vi "FitToolingPinImage.vi"(7 "Pattern Match Settings":T4={"Algorithm"=2, "Number of Matches Requested"=1, "Minimum Match Score"=700.0, "SubPixel Accuracy"=TRUE, "Rotation Angle Ranges"=[{"Start"=-90.0, "End"=90.0}], "Show Search Area"=FALSE, "Show Result"=TRUE} {"Rotation Angle Ranges"."End" format="%.1f"; "Rotation Angle Ranges"."Start" format="%.1f"; "Minimum Match Score" min=0 max=1000 format="%.2f"; "Number of Matches Requested" min=1; "Algorithm" items=["All", "Low Discrepancy Sampling", "Grayscale Value Pyramid", "Gradients Pyramid"]}, 9 "Calibrated Image":T1, 10 "Search Rect":T3={"Left"=0, "Top"=0, "Right"=2147483647, "Bottom"=2147483647, "Rotation"=0.0} {"Rotation" format="%.2f"; "Left" scale=0.0..1024.0; "Right" scale=0.0..1024.0}, 11 "Template":T1) -> (1 "Corner positions":sgl[](array[numeric]), 3 "Refnum out":T1)   [LabVIEW 2016]
uses:
  <vilib>/vision/Image Controls.llb/IMAQ Image.ctl
  <vilib>/vision/NI_Vision_Development_Module.lvlib
panel:
  out "Matches (pixel)":T2(array[cluster]) {"Bounding Box"."y" format="%.2f"; "Bounding Box"."x" format="%.2f"; "Position"."y" format="%.2f"; "Position"."x" format="%.2f"; "Score" format="%.2f"; "Scale" format="%.2f"; "Angle" format="%.2f"}
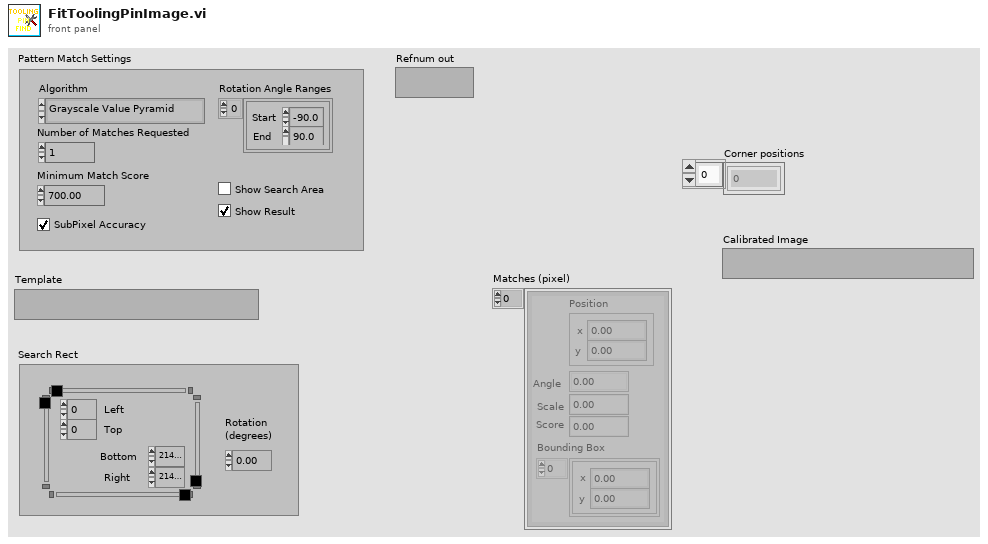
[diagram p1: front panel]
types:
  T1 = typedef "IMAQ Image.ctl" = refnum<image>
  T2 = cluster{"Position":cluster{"x":sgl, "y":sgl}, "Angle":sgl, "Scale":sgl, "Score":sgl, "Bounding Box":cluster{"x":sgl, "y":sgl}[]}[]
  T3 = typedef "IMAQ Rectangle" = cluster{"Left":i32, "Top":i32, "Right":i32, "Bottom":i32, "Rotation":dbl}
  T4 = cluster{"Algorithm":i32, "Number of Matches Requested":i32, "Minimum Match Score":sgl, "SubPixel Accuracy":bool, "Rotation Angle Ranges":cluster{"Start":sgl, "End":sgl}[], "Show Search Area":bool, "Show Result":bool}
  T5 = cluster{"Left":i32, "Top":i32, "Right":i32, "Bottom":i32, "Rotation":dbl}
  T6 = cluster{"Matches (pixel)[0]":cluster{"Position":cluster{"x":sgl, "y":sgl}, "Angle":sgl, "Scale":sgl, "Score":sgl, "Bounding Box":cluster{"x":sgl, "y":sgl}[]}, "Matches (pixel)[1]":cluster{"Position":cluster{"x":sgl, "y":sgl}, "Angle":sgl, "Scale":sgl, "Score":sgl, "Bounding Box":cluster{"x":sgl, "y":sgl}[]}, "Matches (pixel)[2]":cluster{"Position":cluster{"x":sgl, "y":sgl}, "Angle":sgl, "Scale":sgl, "Score":sgl, "Bounding Box":cluster{"x":sgl, "y":sgl}[]}, "Matches (pixel)[3]":cluster{"Position":cluster{"x":sgl, "y":sgl}, "Angle":sgl, "Scale":sgl, "Score":sgl, "Bounding Box":cluster{"x":sgl, "y":sgl}[]}, "Matches (pixel)[4]":cluster{"Position":cluster{"x":sgl, "y":sgl}, "Angle":sgl, "Scale":sgl, "Score":sgl, "Bounding Box":cluster{"x":sgl, "y":sgl}[]}, "Matches (pixel)[5]":cluster{"Position":cluster{"x":sgl, "y":sgl}, "Angle":sgl, "Scale":sgl, "Score":sgl, "Bounding Box":cluster{"x":sgl, "y":sgl}[]}, "Matches (pixel)[6]":cluster{"Position":cluster{"x":sgl, "y":sgl}, "Angle":sgl, "Scale":sgl, "Score":sgl, "Bounding Box":cluster{"x":sgl, "y":sgl}[]}, "Matches (pixel)[7]":cluster{"Position":cluster{"x":sgl, "y":sgl}, "Angle":sgl, "Scale":sgl, "Score":sgl, "Bounding Box":cluster{"x":sgl, "y":sgl}[]}, "Matches (pixel)[8]":cluster{"Position":cluster{"x":sgl, "y":sgl}, "Angle":sgl, "Scale":sgl, "Score":sgl, "Bounding Box":cluster{"x":sgl, "y":sgl}[]}}
  T7 = cluster{"Position":cluster{"x":sgl, "y":sgl}, "Angle":sgl, "Scale":sgl, "Score":sgl, "Bounding Box":cluster{"x":sgl, "y":sgl}[]}
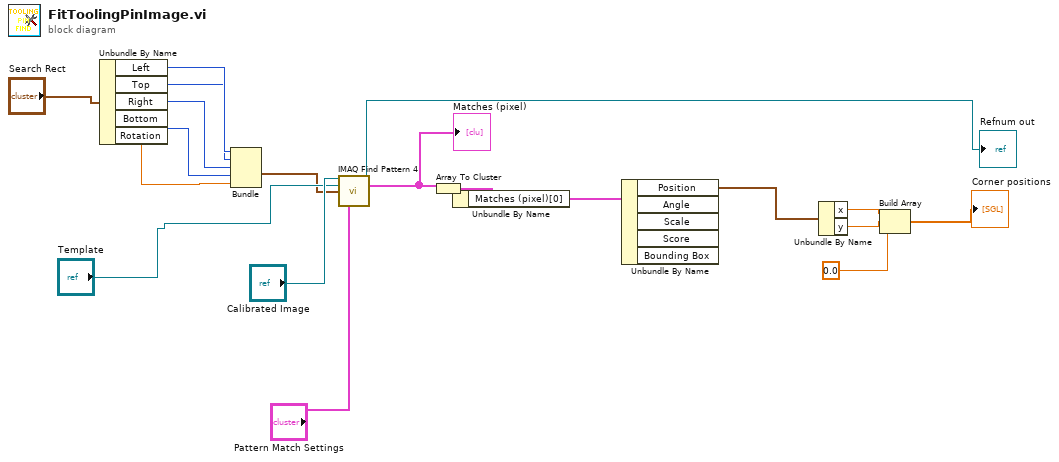
[diagram p0: block diagram]
diagram:
  n1 = Unbundle By Name("Search Rect") -> ("Left"=w18:i32, "Top"=w1:i32, "Right"=w15:i32, "Bottom"=w2:i32, "Rotation"=w14:dbl)
  n2 = Bundle("Left"=w18, "Top"=w1, "Right"=w15, "Bottom"=w2, "Rotation"=w14) -> (w3:T5)  [unwired: 1 in]
  n3 = call "IMAQ Find Pattern 4"("Image"="Calibrated Image", "Template"="Template", "Search Rect"=w3, "Settings"="Pattern Match Settings") -> ("Image Out"=→"Refnum out":T1, "Matches (pixel)"=w12:T2)  [unwired: 5 in, 5 out]
  "Matches (pixel)" <- w12
  n4 = Array To Cluster(array=w12) -> (cluster=w11:T6)
  n5 = Unbundle By Name(w11) -> ("Matches (pixel)[0]"=w10:T7)
  n6 = Unbundle By Name(w10) -> ("Position"=w9:cluster{"x":sgl, "y":sgl})  [unwired: 4 out]
  n7 = Unbundle By Name(w9) -> ("x"=w8:sgl, "y"=w7:sgl)
  n8 = Build Array(w8, w7, sgl 0.0 ("element")) -> (→"Corner positions":sgl[])
